vi "Compile Events.vi"(8 "error in (no error)":errorcluster, 10 "Channel Descriptors in":T1, 11 "Custom Device Ref":T8 format="%.0x") -> (0 "error out":errorcluster, 2 "Channel Descriptors out":T1, 3 "Custom Device Ref dup":T8 format="%.0x")   [LabVIEW 2011, in "Engine Sim System Explorer.lvlib"]
uses:
  Engine Sim System Explorer.lvlib
  <vilib>/NI Veristand/Custom Device API/Custom Device Item Ref.ctl
  Shared/Channel Descriptors.ctl
  Shared/FPGA Write Descriptor.ctl
  Shared/InputChannelTypes.ctl
  <vilib>/rvi/DataTransferAndStorage/Container/Common/niFpgaDataTypeControl.ctl
  Shared/FPGA Read Descriptor.ctl
  Shared/OutputChannelTypes.ctl
  Shared/Status Chan Descriptor.ctl
  Shared/Engine Simulation Global.vi
  <vilib>/NI Veristand/Custom Device Tools/Custom Device Utility Library/NI VeriStand - Search for Item by GUID.vi
  <vilib>/NI Veristand/Custom Device API/Get Item Property (Double).vi
  <vilib>/NI Veristand/Custom Device Tools/Custom Device Utility Library/NI VeriStand - Search for All Items by GUID.vi
  <vilib>/NI Veristand/Custom Device API/Get Item Property (Boolean).vi
  <vilib>/NI Veristand/Custom Device Tools/Custom Device Utility Library/Custom Device Utility Library.lvlib
  Engine Simulation Shared.lvlib
  <vilib>/NI Veristand/Custom Device API/Custom Device API.lvlib
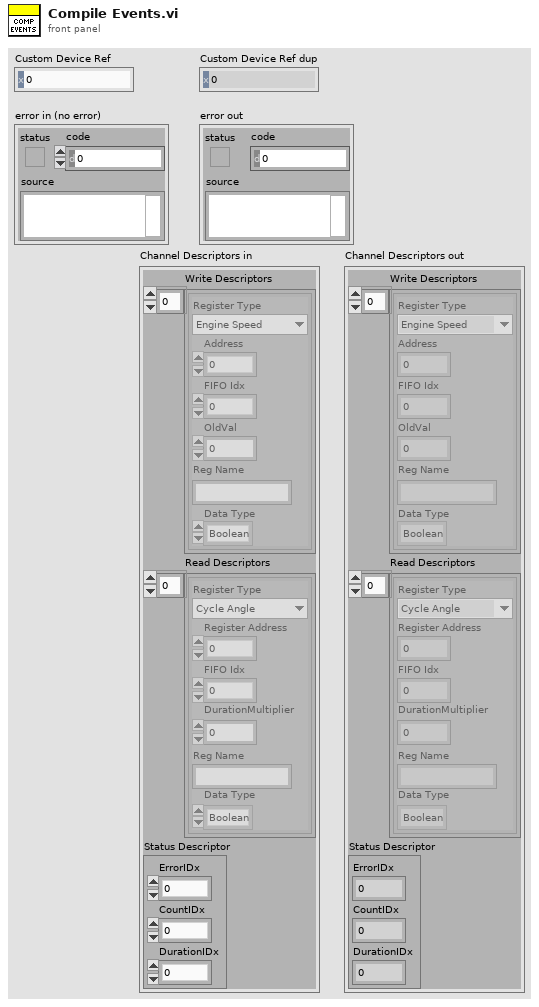
[diagram p1: front panel]
types:
  T1 = typedef "Engine Simulation Shared.lvlib/Channel Descriptors.ctl" = cluster{"Write Descriptors":T2[], "Read Descriptors":T5[], "Status Descriptor":T7}
  T2 = typedef "Engine Simulation Shared.lvlib/FPGA Write Descriptor.ctl" = cluster{"Register Type":T3, "Address":u32, "FIFO Idx":i32, "OldVal":dbl, "Reg Name":string, "Data Type":T4}
  T3 = typedef "Engine Simulation Shared.lvlib/InputChannelTypes.ctl" = enum16{"Engine Speed", "Offset"}
  T4 = typedef "niFpgaDataTypeControl.ctl" = enum32{"Boolean", "I8", "I16", "I32", "I64", "U8", "U16", "U32", "U64", "FXP", "CustomControl"}
  T5 = typedef "Engine Simulation Shared.lvlib/FPGA Read Descriptor.ctl" = cluster{"Register Type":T6, "Register Address":u32, "FIFO Idx":i32, "DurationMultiplier":dbl, "Reg Name":string, "Data Type":T4}
  T6 = typedef "Engine Simulation Shared.lvlib/OutputChannelTypes.ctl" = enum16{"Cycle Angle", "Crank Angle", "Time Duration", "Angle Duration", "Start Angle", "End Angle"}
  T7 = typedef "Engine Simulation Shared.lvlib/Status Chan Descriptor.ctl" = cluster{"ErrorIDx":i32, "CountIDx":i32, "DurationIDx":i32}
  T8 = typedef "Custom Device API.lvlib/Custom Device Item Ref.ctl" = u64
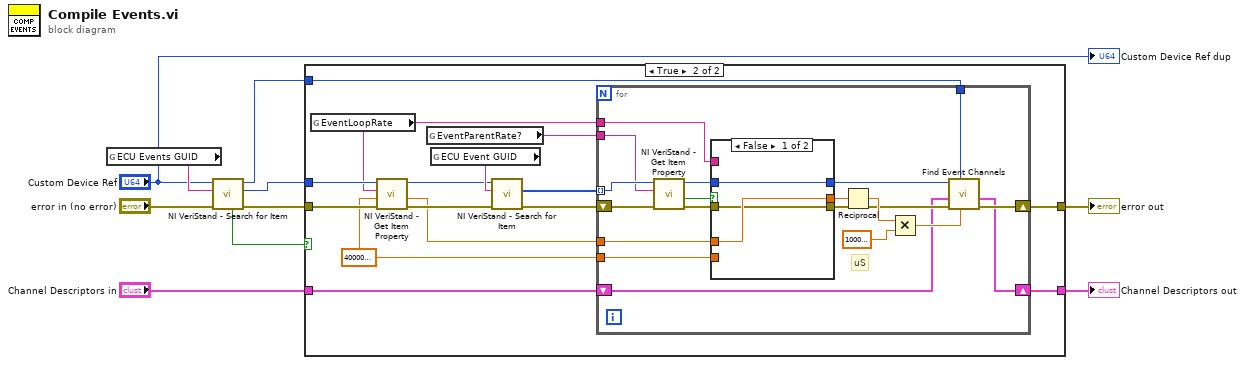
[diagram p0: block diagram]
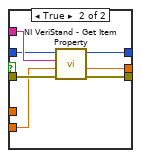
[diagram p3: hidden frame]
diagram:
  n1 = global read "Engine Simulation Global.vi" "ECU Events GUID"() -> (w7:string)
  n2 = call-poly <vilib>:"NI VeriStand - Search for Item.vi"("error in"="error in (no error)", "Item GUID"=w7, "Section Ref in"="Custom Device Ref") -> ("error out"=w8:errorcluster, "Item Ref"=w4:T8, "Section Ref out"=w1:T8, "Found"=w6:bool)  [unwired: 5 in]
  n3 = case shown="True" w6 {
    tunnel: [w12 w24] -> w9
    tunnel: w8 -> [w12 w23]
    tunnel: w4 -> [_ w21]
    tunnel: "Channel Descriptors in" -> [w11 w15]
    tunnel: [w11 w14] -> w2
    tunnel: w1 -> [_ w13]
    frame False {
    }
    frame True {
      w17 = 40000000.0
      n4 = global read "Engine Simulation Global.vi" "EventLoopRate"() -> (w19:string)
      n5 = call-poly <vilib>:"NI VeriStand - Get Item Property.vi"("error in (no error)"=w23, "Default Value"=w17, "Property Name"=w19, "Item Ref in"=w21) -> ("error out"=w22:errorcluster, "Value"=w16:dbl, "Item Ref out"=w20:T8)  [unwired: 4 in, 1 out]
      n6 = global read "Engine Simulation Global.vi" "EventParentRate?"() -> (w18:string)
      n7 = global read "Engine Simulation Global.vi" "ECU Event GUID"() -> (w27:string)
      n8 = call-poly <vilib>:"NI VeriStand - Search for Item.vi"("error in"=w22, "Item GUID"=w27, "Section Ref in"=w20) -> ("error out"=w26:errorcluster, "Item Refs"=w25:T8[])  [unwired: 5 in, 2 out]
      n9 = for {
        shift-right: [w34] -> w24
        shift-left: w26 -> [w45]
        tunnel: w25 -> [w43] mode=indexing
        tunnel: w19 -> [w46]
        tunnel: w18 -> [w41]
        tunnel: w17 -> [w39]
        tunnel: w16 -> [w38]
        shift-right: [w29] -> w14
        shift-left: w15 -> [w30]
        tunnel: w13 -> [w28]
        # "uS"
        n10 = call-poly <vilib>:"NI VeriStand - Get Item Property.vi"("error in (no error)"=w45, "Property Name"=w41, "Item Ref in"=w43) -> ("error out"=w44:errorcluster, "Value"=w40:bool, "Item Ref out"=w42:T8)  [unwired: 5 in, 1 out]
        n11 = case shown="False" w40 {
          tunnel: w46 -> [_ w56]
          tunnel: [w48 w55] -> w33
          tunnel: w44 -> [w48 w54]
          tunnel: w42 -> [w47 w53]
          tunnel: w39 -> [_ w52]
          tunnel: [w49 w51] -> w37
          tunnel: w38 -> [w49 _]
          tunnel: [w47 w50] -> w32
          frame False {
          }
          frame True {
            n12 = call-poly <vilib>:"NI VeriStand - Get Item Property.vi"("error in (no error)"=w54, "Default Value"=w52, "Property Name"=w56, "Item Ref in"=w53) -> ("error out"=w55:errorcluster, "Value"=w51:dbl, "Item Ref out"=w50:T8)  [unwired: 4 in, 1 out]
          }
        }
        n13 = Reciprocal(x=w37) -> (1/x=w36:dbl)
        n14 = Multiply(x=w36, y=1000000.0) -> (x*y=w31:dbl)
        n15 = call "Find Event Channels.vi"("duration multiplier"=w31, "Custom Device Ref"=w28, "error in (no error)"=w33, "Channel Descriptors in"=w30, "Event ref"=w32) -> ("error out"=w34:errorcluster, "Channel Descriptors out"=w29:T1)  [unwired: 5 in]
      }
    }
  }
  "error out" <- w9
  "Channel Descriptors out" <- w2
  "Custom Device Ref dup" <- "Custom Device Ref"
